vi "Create Default Line.vi"(10 "Line Name":string) -> (2 "Default Line":T1)   [LabVIEW 2015, in "PID Module configuration.lvclass"]
uses:
  PID Module configuration.lvclass
  Line.ctl
  <vilib>/NI/Tag Bus Module Framework/channel/TBM channel.lvclass
  String Parameters.ctl
  <vilib>/NI/Tag Bus Module Framework/channel/channel classification.ctl
  <vilib>/NI/Tag Bus/tag/Data Type.ctl
  <vilib>/NI/Tag Bus/tag/default value polymorphs/write default value Double.vi
  <vilib>/NI/Tag Bus/tag/tag descriptor.lvclass
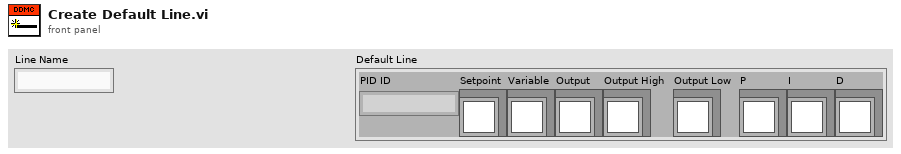
[diagram p1: front panel]
types:
  T1 = typedef "PID Module configuration.lvclass/Line.ctl" = cluster{"PID ID":string, "Setpoint":refnum<class "TBM channel.lvclass">, "Variable":refnum<class "TBM channel.lvclass">, "Output":refnum<class "TBM channel.lvclass">, "Output High":refnum<class "TBM channel.lvclass">, "Output Low":refnum<class "TBM channel.lvclass">, "P":refnum<class "TBM channel.lvclass">, "I":refnum<class "TBM channel.lvclass">, "D":refnum<class "TBM channel.lvclass">}
  T2 = typedef "tag bus.lvlib/tag descriptor.lvclass/Data Type.ctl" = enum16{"Double", "Single", "I64", "I32", "I16", "I8", "U64", "U32", "U16", "U8", "Boolean", "String", "Array of Double", "Array of Single", "Array of I64", "Array of I32", "Array of I16", "Array of I8", "Array of U64", "Array of U32", "Array of U16", "Array of U8", "Array of Boolean", "Array of String"}
  T3 = typedef "PID Module configuration.lvclass/String Parameters.ctl" = enum16{"Setpoint", "Process Variable", "Output", "Proportional Gain", "Integral Time", "Derivative Time", "Range High", "Range Low"}
  T4 = typedef "TBM channel.lvclass/channel classification.ctl" = enum16{"input data", "output data", "processing parameter", "processing result"}
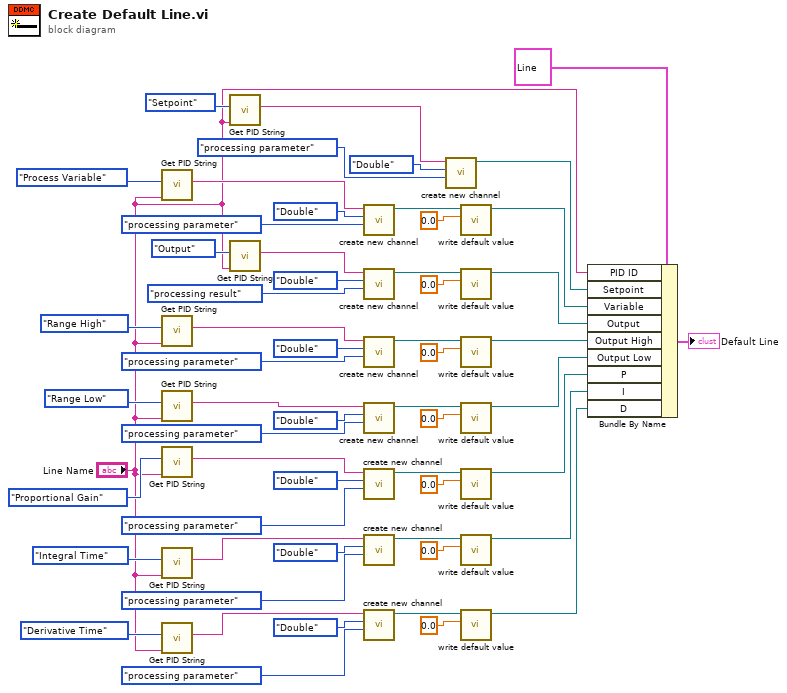
[diagram p0: block diagram]
diagram:
  n1 = call "Get PID String.vi"("PID Loop ID"="Line Name", "PID Parameter"=String_Parameters."Process Variable") -> ("Parameter String"=w49:string)  [unwired: 7 in]
  n2 = call "Get PID String.vi"("PID Loop ID"="Line Name", "PID Parameter"=String_Parameters."Range High") -> ("Parameter String"=w41:string)  [unwired: 7 in]
  n3 = call "Get PID String.vi"("PID Loop ID"="Line Name", "PID Parameter"=String_Parameters."Range Low") -> ("Parameter String"=w36:string)  [unwired: 7 in]
  n4 = call "Get PID String.vi"("PID Loop ID"="Line Name", "PID Parameter"=String_Parameters."Proportional Gain") -> ("Parameter String"=w33:string)  [unwired: 7 in]
  n5 = call "Get PID String.vi"("PID Loop ID"="Line Name", "PID Parameter"=String_Parameters."Integral Time") -> ("Parameter String"=w28:string)  [unwired: 7 in]
  n6 = call "Get PID String.vi"("PID Loop ID"="Line Name", "PID Parameter"=String_Parameters."Derivative Time") -> ("Parameter String"=w25:string)  [unwired: 7 in]
  n7 = call "Get PID String.vi"("PID Loop ID"="Line Name", "PID Parameter"=String_Parameters."Setpoint") -> ("Parameter String"=w52:string)  [unwired: 7 in]
  n8 = call "Get PID String.vi"("PID Loop ID"="Line Name", "PID Parameter"=String_Parameters."Output") -> ("Parameter String"=w44:string)  [unwired: 7 in]
  n9 = call <vilib>:"create new channel.vi"("channel classification"=channel_classification."processing parameter", "data type"=Data_Type."Double", "channel name"=w49) -> ("channel"=w6:refnum<class "TBM channel.lvclass">)  [unwired: 8 in]
  n10 = call <vilib>:"create new channel.vi"("channel classification"=channel_classification."processing result", "data type"=Data_Type."Double", "channel name"=w44) -> ("channel"=w4:refnum<class "TBM channel.lvclass">)  [unwired: 8 in]
  n11 = call <vilib>:"create new channel.vi"("channel classification"=channel_classification."processing parameter", "data type"=Data_Type."Double", "channel name"=w41) -> ("channel"=w2:refnum<class "TBM channel.lvclass">)  [unwired: 8 in]
  n12 = call <vilib>:"create new channel.vi"("channel classification"=channel_classification."processing parameter", "data type"=Data_Type."Double", "channel name"=w36) -> ("channel"=w14:refnum<class "TBM channel.lvclass">)  [unwired: 8 in]
  n13 = call <vilib>:"create new channel.vi"("channel classification"=channel_classification."processing parameter", "data type"=Data_Type."Double", "channel name"=w33) -> ("channel"=w16:refnum<class "TBM channel.lvclass">)  [unwired: 8 in]
  n14 = call <vilib>:"create new channel.vi"("channel classification"=channel_classification."processing parameter", "data type"=Data_Type."Double", "channel name"=w28) -> ("channel"=w11:refnum<class "TBM channel.lvclass">)  [unwired: 8 in]
  n15 = call <vilib>:"create new channel.vi"("channel classification"=channel_classification."processing parameter", "data type"=Data_Type."Double", "channel name"=w25) -> ("channel"=w21:refnum<class "TBM channel.lvclass">)  [unwired: 8 in]
  n16 = call <vilib>:"create new channel.vi"("channel classification"=channel_classification."processing parameter", "data type"=Data_Type."Double", "channel name"=w52) -> ("channel"=w54:refnum<class "TBM channel.lvclass">)  [unwired: 8 in]
  n17 = call-poly <vilib>:"write default value.vi"("default value"=0.0, "system tag in"=w6) -> ("system tag out"=w5:refnum<class "TBM channel.lvclass">)  [unwired: 8 in, 1 out]
  n18 = call-poly <vilib>:"write default value.vi"("default value"=0.0, "system tag in"=w4) -> ("system tag out"=w3:refnum<class "TBM channel.lvclass">)  [unwired: 8 in, 1 out]
  n19 = call-poly <vilib>:"write default value.vi"("default value"=0.0, "system tag in"=w2) -> ("system tag out"=w1:refnum<class "TBM channel.lvclass">)  [unwired: 8 in, 1 out]
  n20 = call-poly <vilib>:"write default value.vi"("default value"=0.0, "system tag in"=w14) -> ("system tag out"=w13:refnum<class "TBM channel.lvclass">)  [unwired: 8 in, 1 out]
  n21 = call-poly <vilib>:"write default value.vi"("default value"=0.0, "system tag in"=w16) -> ("system tag out"=w12:refnum<class "TBM channel.lvclass">)  [unwired: 8 in, 1 out]
  n22 = call-poly <vilib>:"write default value.vi"("default value"=0.0, "system tag in"=w11) -> ("system tag out"=w10:refnum<class "TBM channel.lvclass">)  [unwired: 8 in, 1 out]
  n23 = call-poly <vilib>:"write default value.vi"("default value"=0.0, "system tag in"=w21) -> ("system tag out"=w20:refnum<class "TBM channel.lvclass">)  [unwired: 8 in, 1 out]
  n24 = Bundle By Name(cluster=T1 {"PID ID"="", "Setpoint"=refnum, "Variable"=refnum, "Output"=refnum, "Output High"=refnum, "Output Low"=refnum, "P"=refnum, "I"=refnum, "D"=refnum} ("Line"), "PID ID"="Line Name", "Setpoint"=w54, "Variable"=w5, "Output"=w3, "Output High"=w1, "Output Low"=w13, "P"=w12, "I"=w10, "D"=w20) -> (→"Default Line":T1)
